vi "Initialize.vi"(8 "error in":errorcluster, 11 "Plugin in":refnum<class "MP750510.lvclass">) -> (0 "error out":errorcluster, 3 "Plugin out":refnum<class "MP750510.lvclass">)   [LabVIEW 2025, in "MP750510.lvlib" / "MP750510.lvclass"]
uses:
  MP750510.lvclass
  C:/Program Files/National Instruments/LabVIEW 2025/vi.lib/FlexLogger/SDK/PluginSDK.lvlibp/PEFClasses/SDK/Plugin/Plugin.lvclass
  <vilib>/FlexLogger/SDK/PluginSDK.lvlibp/PEFClasses/SDK/Processing Element/Timing Parameters.ctl
  <vilib>/FlexLogger/SDK/PluginSDK.lvlibp/PEFClasses/SDK/Processing Element/Timing Method.ctl
  <vilib>/FlexLogger/SDK/PluginSDK.lvlibp/PEFClasses/SDK/Setpoint Consumer Channel/Setpoint Consumer Channel.lvclass
  C:/Program Files/National Instruments/LabVIEW 2025/vi.lib/FlexLogger/SDK/PluginSDK.lvlibp/PEFClasses/SDK/Channel/Channel.lvclass
  <vilib>/FlexLogger/SDK/PluginSDK.lvlibp/PEFClasses/SDK/Plugin/ParameterAccess/Write String.vi
  <vilib>/FlexLogger/SDK/PluginSDK.lvlibp/PEFClasses/SDK/Setpoint Consumer Channel/Create Setpoint Consumer Channel.vi
  <vilib>/FlexLogger/SDK/PluginSDK.lvlibp/PEFClasses/SDK/Channel/ParameterAccess/Write Enum.vi
  <vilib>/FlexLogger/SDK/PluginSDK.lvlibp/PEFClasses/SDK/Plugin/Plugin.lvclass
  <vilib>/FlexLogger/SDK/PluginSDK.lvlibp/PEFClasses/SDK/Processing Element/Processing Element.lvclass
  <vilib>/FlexLogger/SDK/PluginSDK.lvlibp/PEFClasses/SDK/Channel/Channel.lvclass
  <vilib>/FlexLogger/SDK/PluginSDK.lvlibp
  C:/Program Files/National Instruments/LabVIEW 2025/vi.lib/FlexLogger/SDK/PluginSDK.lvlibp/PEFClasses/SDK/Consumer Channel/Consumer Channel.lvclass
  C:/Program Files/National Instruments/LabVIEW 2025/vi.lib/FlexLogger/SDK/PluginSDK.lvlibp/PEFClasses/SDK/Setpoint Consumer Channel/Setpoint Consumer Channel.lvclass
  C:/Program Files/National Instruments/LabVIEW 2025/vi.lib/FlexLogger/SDK/PluginSDK.lvlibp/PEFClasses/SDK/Processing Element/Processing Element.lvclass
  C:/Users/Steve/Documents/Git/MP750510_Plugin/FlexLogger/MP750510 - Copy/MP750510.lvclass
panel:
  out "Array":string[](array[string])
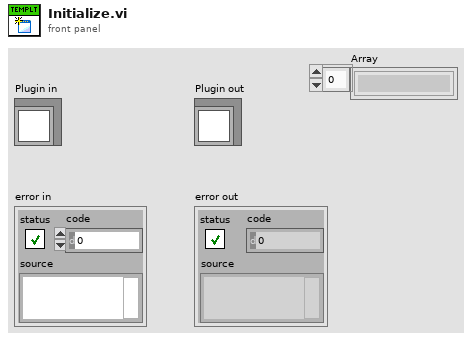
[diagram p1: front panel]
types:
  T1 = typedef "PluginSDK.lvlibp/Processing Element.lvclass/Timing Parameters.ctl" = cluster{"Timing Method":T2, "Timing Period (ms)":i32}
  T2 = typedef "PluginSDK.lvlibp/Processing Element.lvclass/Timing Method.ctl" = enum16{"Periodic", "Immediate", "On Data Ready", "Triggered"}
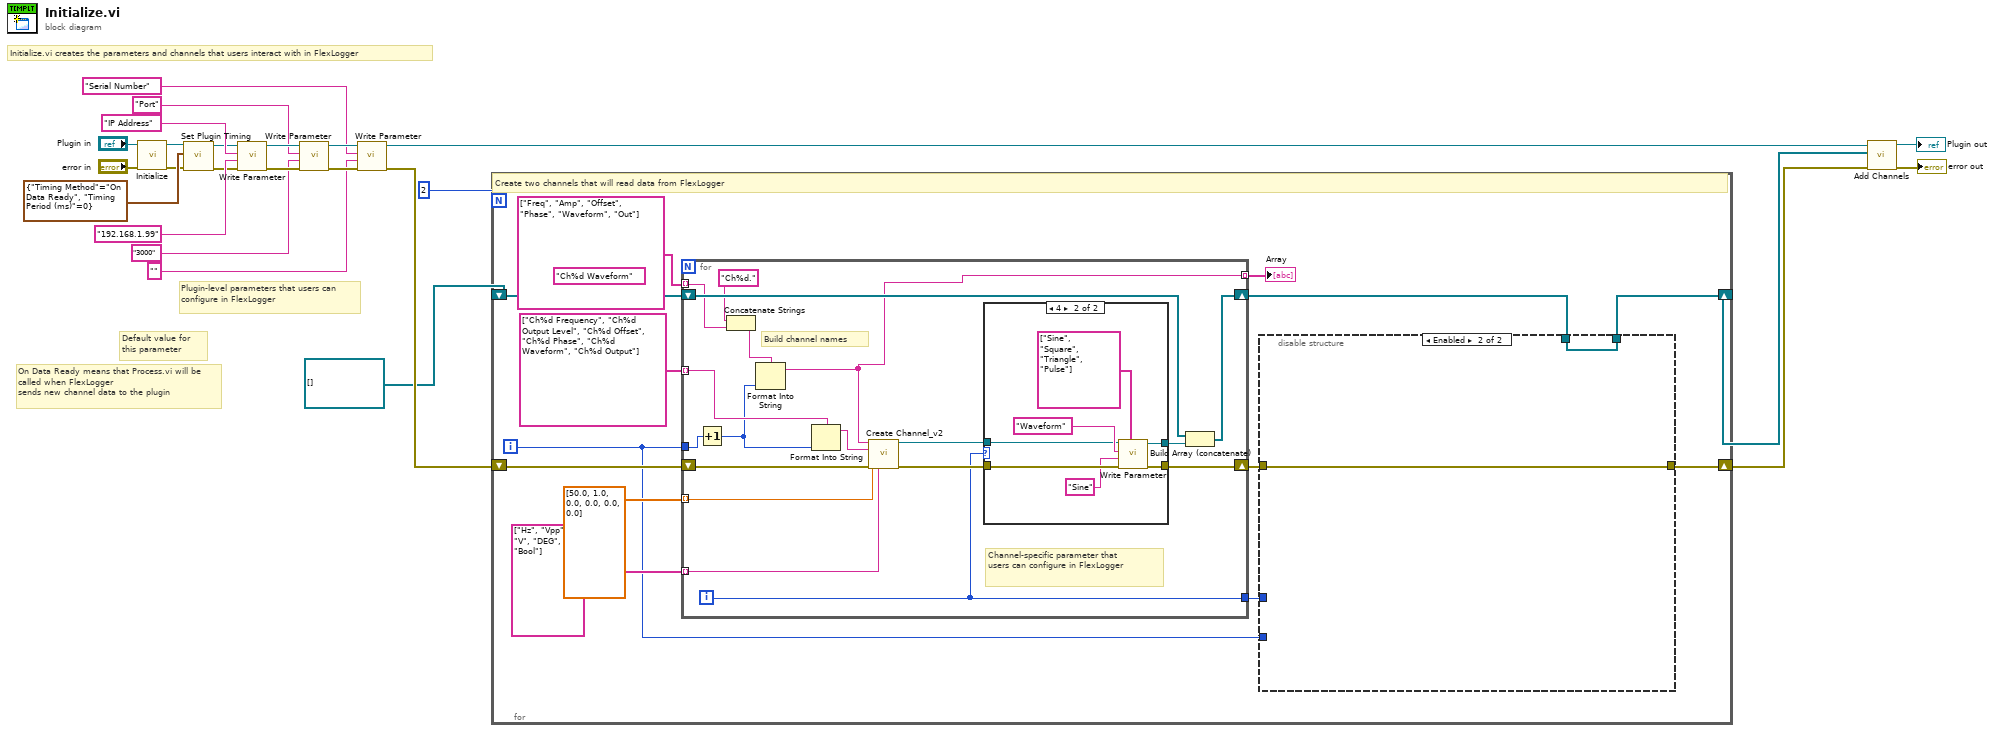
[diagram p0: block diagram]
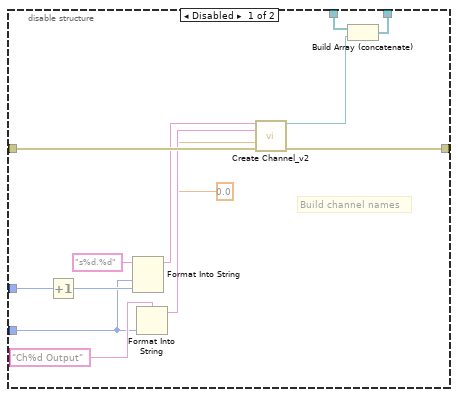
[diagram p2: hidden frame]
diagram:
  # "Default value for this parameter"
  # "Plugin-level parameters that users can configure in FlexLogger"
  # "On Data Ready means that Process.vi will be called when FlexLogger \nsends new channel data to the plugin"
  # "Initialize.vi creates the parameters and channels that users interact with in FlexLogger"
  n1 = call-parent "Initialize.vi"("error in (no error)"="error in", "Plugin in"="Plugin in") -> ("error out"=w14:errorcluster, "Plugin out"=w13:refnum<class "MP750510.lvclass">)  [unwired: 8 in]
  n2 = call <vilib>:"Set Plugin Timing.vi"("error in (no error)"=w14, "Timing Parameters"=T1 {"Timing Method"=enum."On Data Ready", "Timing Period (ms)"=0}, "Plugin in"=w13) -> ("error out"=w11:errorcluster, "Plugin out"=w12:refnum<class "MP750510.lvclass">)  [unwired: 7 in]
  n3 = call-poly <vilib>:"Write Parameter.vi"("error in (no error)"=w11, "Value"="192.168.1.99", "Name"="IP Address", "Plugin in"=w12) -> ("error out"=w17:errorcluster, "Plugin out"=w16:refnum<class "MP750510.lvclass">)  [unwired: 6 in]
  n4 = call-poly <vilib>:"Write Parameter.vi"("error in (no error)"=w17, "Value"="3000", "Name"="Port", "Plugin in"=w16) -> ("error out"=w8:errorcluster, "Plugin out"=w6:refnum<class "MP750510.lvclass">)  [unwired: 6 in]
  n5 = call-poly <vilib>:"Write Parameter.vi"("error in (no error)"=w8, "Value"="", "Name"="Serial Number", "Plugin in"=w6) -> ("error out"=w7:errorcluster, "Plugin out"=w5:refnum<class "MP750510.lvclass">)  [unwired: 6 in]
  n6 = for {
    N: 2 -> [_]
    shift-right: [w28] -> w20
    shift-left: w7 -> [w38]
    shift-right: [w31] -> w1
    shift-left: refnum<class "Setpoint Consumer Channel.lvclass">[] [] -> [w32]
    i -> [w29]
    (unwired) "Ch%d Waveform" ("format string")
    # "Create two channels that will read data from FlexLogger"
    n7 = for {
      tunnel: w29 -> [w58]
      tunnel: string[] ["Ch%d Frequency", "Ch%d Output Level", "Ch%d Offset", "Ch%d Phase", "Ch%d Waveform", "Ch%d Output"] -> [w66] mode=indexing
      shift-right: [w70] -> w34
      shift-left: w38 -> [w68]
      tunnel: string[] ["Hz", "Vpp", "V", "DEG", "", "Bool"] -> [w65] mode=indexing
      tunnel: dbl[] [50.0, 1.0, 0.0, 0.0, 0.0, 0.0] -> [w64] mode=indexing
      shift-right: [w62] -> w33
      shift-left: w32 -> [w61]
      tunnel: [w60] -> w30
      tunnel: string[] ["Freq", "Amp", "Offset", "Phase", "Waveform", "Out"] -> [w59] mode=indexing
      tunnel: [w54] -> w26 mode=indexing
      i -> [w60]
      # "Build channel names"
      # "Channel-specific parameter that users can configure in FlexLogger"
      n8 = Increment(x=w58) -> (x+1=w57:i32)
      n9 = Concatenate Strings("Ch%d." ("format string"), w59) -> (w55:string)
      n10 = Format Into String(format string=w55, w57) -> (resulting string=w54:string)  [unwired: 2 in, 1 out]
      n11 = Format Into String(format string=w66, w57) -> (resulting string=w71:string)  [unwired: 2 in, 1 out]
      n12 = call-poly <vilib>:"Create Channel_v2.vi"("Unique Channel Identifier"=w54, "Default Channel Name"=w71, "Default Value"=w64, "error in (no error)"=w68, "Unit"=w65) -> ("Setpoint Consumer Channel"=w69:refnum<class "Setpoint Consumer Channel.lvclass">, "error out"=w67:errorcluster)  [unwired: 9 in]
      n13 = case shown="4" w60 {
        tunnel: [w72 w79] -> w70
        tunnel: w69 -> [w73 w78]
        tunnel: [w73 w77] -> w63
        tunnel: w67 -> [w72 w76]
        frame Default {
        }
        frame 4 {
          n14 = call-poly <vilib>:"Write Parameter.vi"("Possible Values"=string[] ["Sine", "Square", "Triangle", "Pulse"], "error in (no error)"=w76, "Current Value"="Sine" ("format string"), "Name"="Waveform", "Channel in"=w78) -> ("error out"=w79:errorcluster, "Channel out"=w77:refnum<class "Setpoint Consumer Channel.lvclass">)  [unwired: 5 in]
        }
      }
      n15 = Build Array (concatenate)(w61, w63) -> (w62:refnum<class "Setpoint Consumer Channel.lvclass">[])
    }
    "Array" <- w26
    n16 = disable-structure shown="Enabled" {
      disable-tunnel: w34 -> [w51 w53]
      disable-tunnel: w33 -> [w50 w52]
      disable-tunnel: [w49 w52] -> w31
      disable-tunnel: w30 -> [w48 _]
      disable-tunnel: w29 -> [w43 _]
      disable-tunnel: [w40 w53] -> w28
      frame Disabled {
        # "Build channel names"
        n17 = Increment(x=w48) -> (x+1=w46:i32)
        n18 = Format Into String(format string="s%d.%d", w43, w46) -> (resulting string=w45:string)  [unwired: 2 in, 1 out]
        n19 = Format Into String(format string="Ch%d Output", w43) -> (resulting string=w42:string)  [unwired: 2 in, 1 out]
        n20 = call-poly <vilib>:"Create Channel_v2.vi"("Unique Channel Identifier"=w45, "Default Channel Name"=w42, "Default Value"=0.0, "error in (no error)"=w51) -> ("Setpoint Consumer Channel"=w39:refnum<class "Setpoint Consumer Channel.lvclass">, "error out"=w40:errorcluster)  [unwired: 10 in]
        n21 = Build Array (concatenate)(w50, w39) -> (w49:refnum<class "Setpoint Consumer Channel.lvclass">[])
      }
      frame Enabled {
      }
    }
  }
  n22 = call <vilib>:"Add Channels.vi"("error in (no error)"=w20, "Channels"=w1, "Plugin in"=w5) -> ("error out"=→"error out":errorcluster, "Plugin out"=→"Plugin out":refnum<class "MP750510.lvclass">)  [unwired: 7 in]
